vi "read_raw_data.vi"() -> ()   [LabVIEW 2017]
uses:
  <vilib>/Utility/file.llb/Write Delimited Spreadsheet (I64).vi
panel:
  out "file path (dialog if empty) 2":path
  out "ip":u64 format="%x"
  out "data 9":string
  out "result string":string
  out "sent number":u64 format="%x"
  out "trigger number":u64 format="%x"
  out "data 8":string
  out "data 7":string
  out "data":u64[](array[numeric]) format="%x"
  out "data 2":string
  out "data 4":string
  out "coarse time":u64 format="%x"
  out "error out":errorcluster
  out "substring":string
  out "number 3":u32
  out "channel number":u64 format="%x"
  in  "channel":u64
  out "data 6":string
  out "data 3":string
  in  "file (use dialog)":path
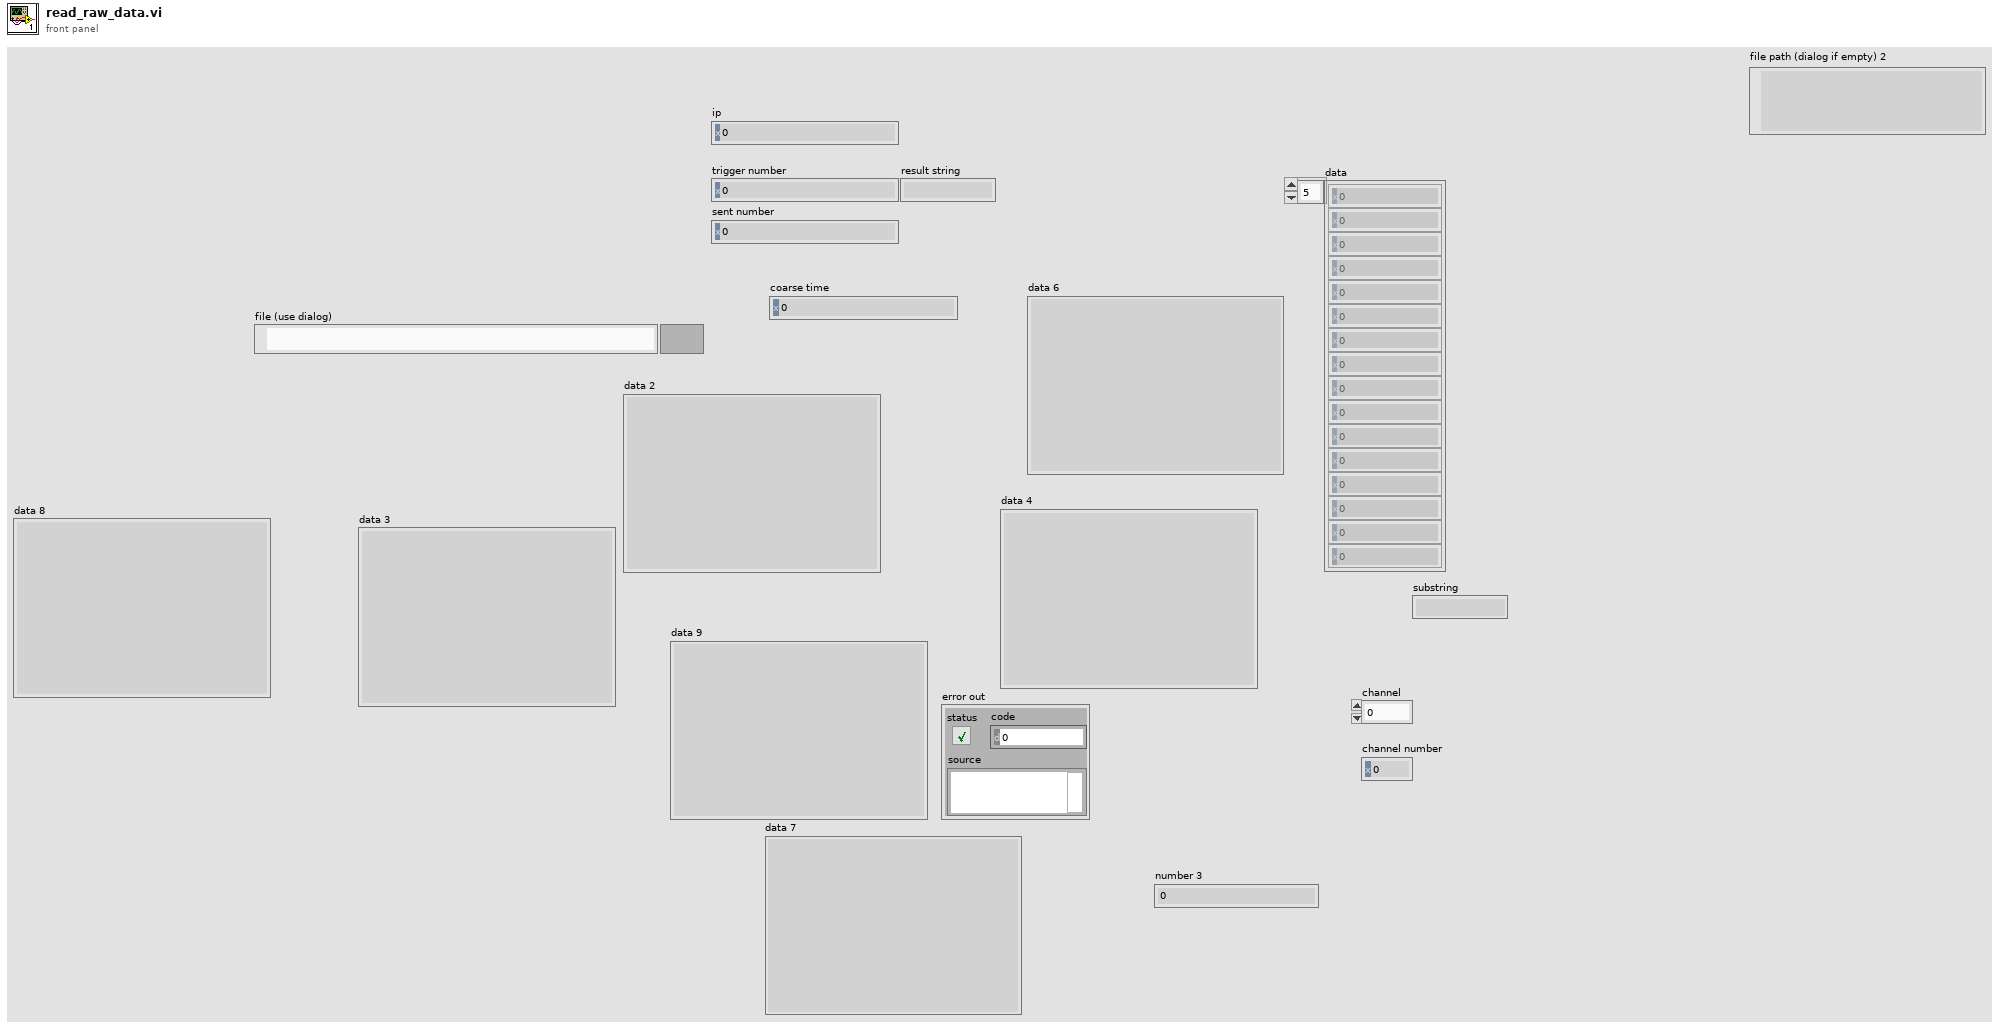
[diagram p1: front panel]
types:
  T1 = enum16{"open", "replace", "create", "open or create", "replace or create", "replace or create with confirmation"}
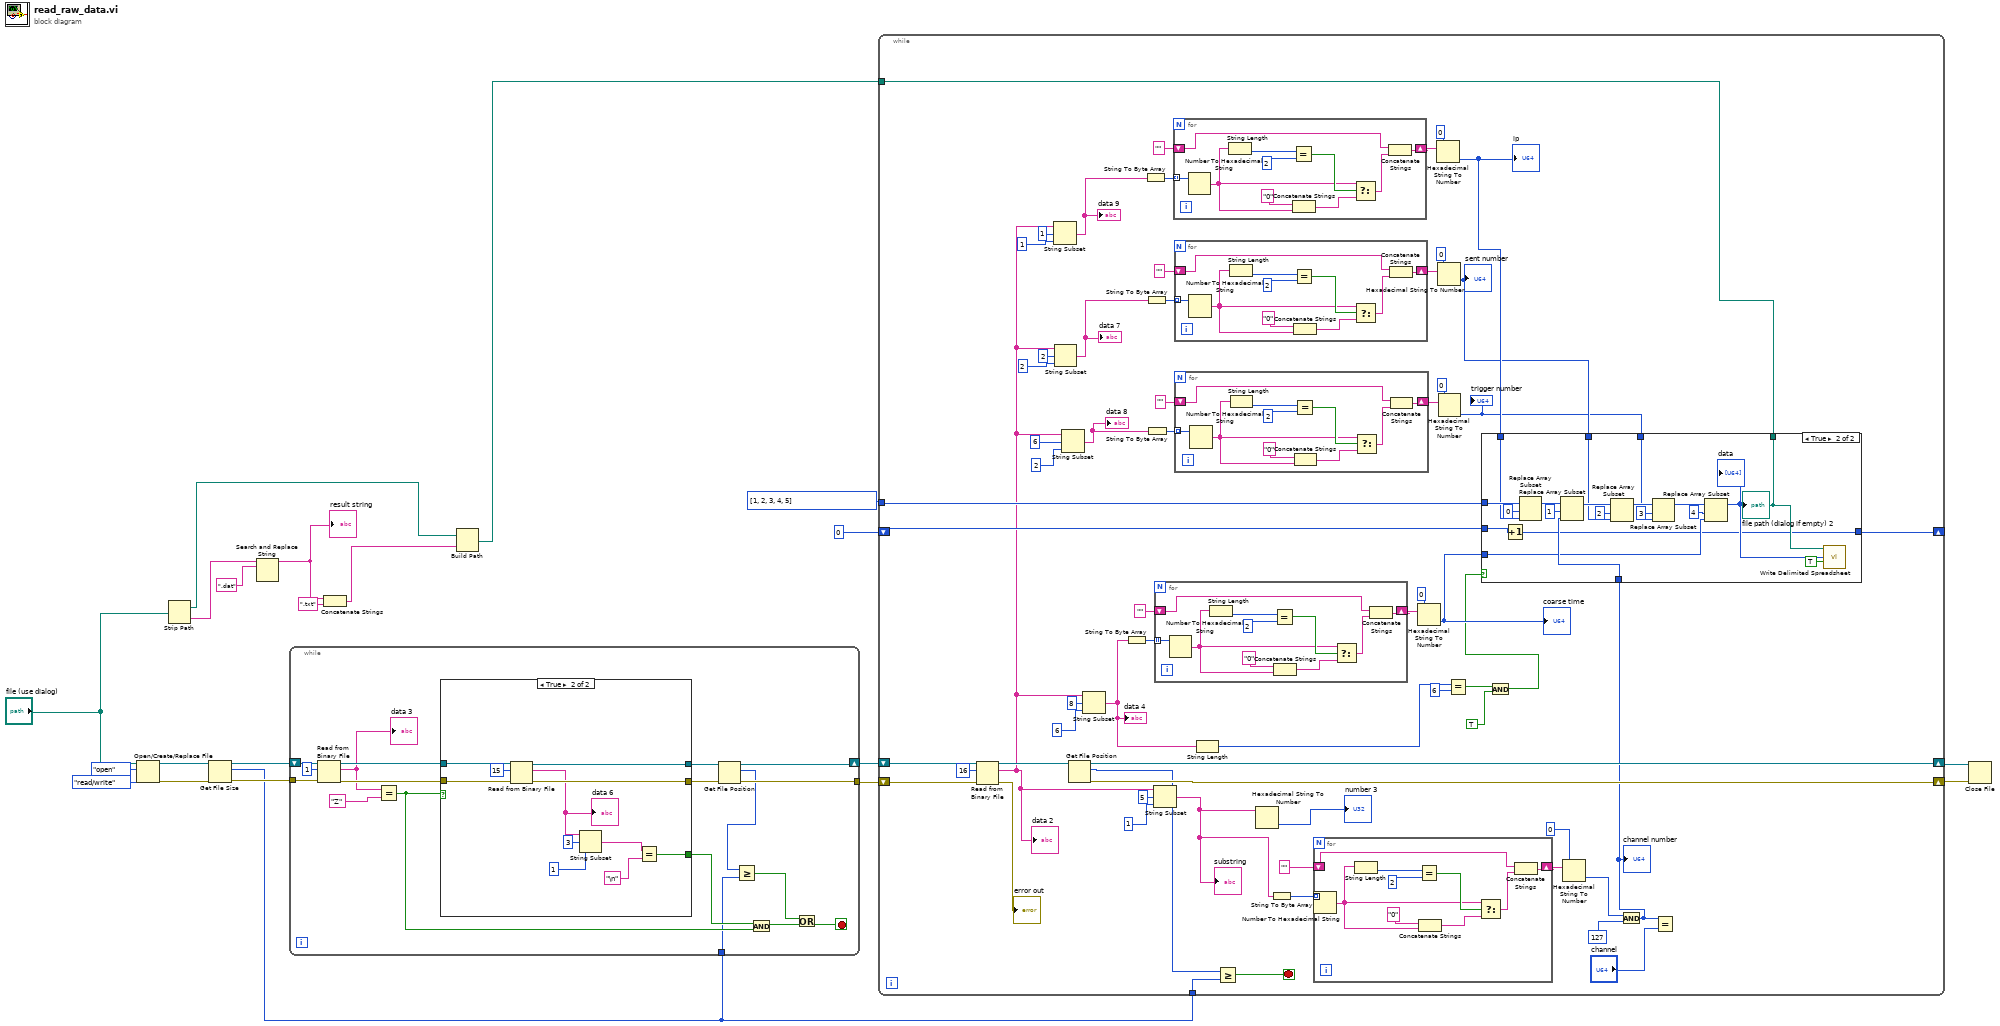
[diagram p0: block diagram]
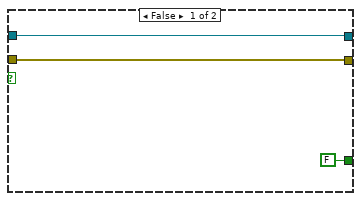
[diagram p3: hidden frame]
diagram:
  n1 = Open/Create/Replace File(file path (use dialog)="file (use dialog)", operation (0:open)=T1."open", access (0:read/write)=enum16{"read/write", "read-only", "write-only"}."read/write") -> (refnum out=w21:refnum<file>, error out=w15:errorcluster)  [unwired: 3 in, 1 out]
  n2 = Strip Path(path="file (use dialog)") -> (stripped path=w2:path, name=w7:string)
  n3 = Get File Size(file=w21, error in=w15) -> (refnum out=w16:refnum<file>, size (in bytes)=w9:i64, 0:w14:errorcluster)
  n4 = Search and Replace String(input string=w7, search string=".dat") -> (result string=w5:string)  [unwired: 6 in, 3 out]
  "result string" <- w5
  n5 = while {
    tunnel: w14 -> [w38]
    shift-right: [w26] -> w17
    shift-left: w16 -> [w39]
    tunnel: [w27] -> w18
    tunnel: w9 -> [w25]
    stop <- w23 stop-if-true
    n6 = Read from Binary File(8:w38, 10:1 ("count (1)"), 11:w39) -> (0:w34:errorcluster, 2:w32:string, 3:w35:refnum<file>)  [unwired: 3 in, 1 out]
    "data 3" <- w32
    n7 = Equal?(x=w32, y="Z") -> (x = y?=w29:bool)
    n8 = case shown="True" w29 {
      tunnel: w35 -> [w42 w53]
      tunnel: w34 -> [w41 w52]
      tunnel: [w42 w50] -> w33
      tunnel: [w41 w49] -> w28
      tunnel: [FALSE w43] -> w30
      frame False {
      }
      frame True {
        n9 = Read from Binary File(8:w52, 10:15 ("count (1)"), 11:w53) -> (0:w49:errorcluster, 2:w46:string, 3:w50:refnum<file>)  [unwired: 3 in, 1 out]
        "data 6" <- w46
        n10 = String Subset(string=w46, offset (0)=3, length (rest)=1 ("length (rest)")) -> (substring=w45:string)
        n11 = Equal?(x=w45, y="\n") -> (x = y?=w43:bool)
      }
    }
    n12 = Get File Position(4:w28, 7:w33) -> (0:w27:errorcluster, 2:w24:i64, 3:w26:refnum<file>)
    n13 = Greater Or Equal?(x=w24, y=w25) -> (x >= y?=w22:bool)
    n14 = Compound Arithmetic op=AND(w30, w29) -> (w31:bool)
    n15 = Or(x=w22, y=w31) -> (x .or. y?=w23:bool)
  }
  n16 = Concatenate Strings(w5, ".txt" ("string")) -> (w3:string)
  n17 = Build Path(base path=w2, name or relative path=w3) -> (appended path=w1:path)
  n18 = while {
    shift-right: [w112] -> w13
    shift-left: w17 -> [w116]
    shift-right: [w114] -> w12
    shift-left: w18 -> [w117]
    tunnel: w9 -> [w110]
    shift-right: [w54] -> _
    shift-left: 0 ("length (rest)") -> [w89]
    tunnel: w1 -> [w55]
    tunnel: u64[] [1, 2, 3, 4, 5] -> [w88]
    stop <- w109 stop-if-true
    n19 = Read from Binary File(8:w117, 10:16 ("count (1)"), 11:w116) -> (0:→"error out":errorcluster, 2:w60:string, 3:w113:refnum<file>)  [unwired: 3 in, 1 out]
    "data 2" <- w60
    n20 = String Subset(string=w60, offset (0)=1, length (rest)=1 ("length (rest)")) -> (substring=w67:string)
    "data 9" <- w67
    n21 = String Subset(string=w60, offset (0)=2, length (rest)=2 ("length (rest)")) -> (substring=w69:string)
    "data 7" <- w69
    n22 = String Subset(string=w60, offset (0)=6, length (rest)=2 ("length (rest)")) -> (substring=w74:string)
    "data 8" <- w74
    n23 = Get File Position(7:w113) -> (0:w114:errorcluster, 2:w111:i64, 3:w112:refnum<file>)  [unwired: 1 in]
    n24 = String Subset(string=w60, offset (0)=8, length (rest)=6 ("length (rest)")) -> (substring=w85:string)
    "data 4" <- w85
    n25 = String To Byte Array(string=w85) -> (unsigned byte array=w105:u8[])
    n26 = String To Byte Array(string=w67) -> (unsigned byte array=w64:u8[])
    n27 = String To Byte Array(string=w69) -> (unsigned byte array=w72:u8[])
    n28 = String To Byte Array(string=w74) -> (unsigned byte array=w76:u8[])
    n29 = String Subset(string=w60, offset (0)=5, length (rest)=1 ("length (rest)")) -> (substring=w92:string)
    "substring" <- w92
    n30 = for {
      shift-right: [w187] -> w104
      shift-left: "" ("format string") -> [w184]
      tunnel: w105 -> [w188] mode=indexing
      n31 = Number To Hexadecimal String(2:w188) -> (0:w180:string)  [unwired: 1 in]
      n32 = String Length(string=w180) -> (length=w186:i32)
      n33 = Equal?(x=w186, y=2) -> (x = y?=w183:bool)
      n34 = Concatenate Strings("0" ("format string"), w180) -> (w182:string)
      n35 = Select(t=w180, s=w183, f=w182) -> (s? t:f=w179:string)
      n36 = Concatenate Strings(w184, w179) -> (w187:string)
    }
    n37 = for {
      shift-right: [w126] -> w65
      shift-left: "" ("format string") -> [w123]
      tunnel: w64 -> [w127] mode=indexing
      n38 = Number To Hexadecimal String(2:w127) -> (0:w119:string)  [unwired: 1 in]
      n39 = String Length(string=w119) -> (length=w125:i32)
      n40 = Equal?(x=w125, y=2) -> (x = y?=w122:bool)
      n41 = Concatenate Strings("0" ("format string"), w119) -> (w121:string)
      n42 = Select(t=w119, s=w122, f=w121) -> (s? t:f=w118:string)
      n43 = Concatenate Strings(w123, w118) -> (w126:string)
    }
    n44 = for {
      shift-right: [w136] -> w71
      shift-left: "" ("format string") -> [w133]
      tunnel: w72 -> [w137] mode=indexing
      n45 = Number To Hexadecimal String(2:w137) -> (0:w129:string)  [unwired: 1 in]
      n46 = String Length(string=w129) -> (length=w135:i32)
      n47 = Equal?(x=w135, y=2) -> (x = y?=w132:bool)
      n48 = Concatenate Strings("0" ("format string"), w129) -> (w131:string)
      n49 = Select(t=w129, s=w132, f=w131) -> (s? t:f=w128:string)
      n50 = Concatenate Strings(w133, w128) -> (w136:string)
    }
    n51 = for {
      shift-right: [w146] -> w77
      shift-left: "" ("format string") -> [w143]
      tunnel: w76 -> [w147] mode=indexing
      n52 = Number To Hexadecimal String(2:w147) -> (0:w139:string)  [unwired: 1 in]
      n53 = String Length(string=w139) -> (length=w145:i32)
      n54 = Equal?(x=w145, y=2) -> (x = y?=w142:bool)
      n55 = Concatenate Strings("0" ("format string"), w139) -> (w141:string)
      n56 = Select(t=w139, s=w142, f=w141) -> (s? t:f=w138:string)
      n57 = Concatenate Strings(w143, w138) -> (w146:string)
    }
    n58 = String Length(string=w85) -> (length=w83:i32)
    n59 = Greater Or Equal?(x=w111, y=w110) -> (x >= y?=w109:bool)
    n60 = Hexadecimal String To Number(string=w92) -> (number=→"number 3":u32)  [unwired: 2 in, 1 out]
    n61 = String To Byte Array(string=w92) -> (unsigned byte array=w95:u8[])
    n62 = for {
      shift-right: [w177] -> w94
      shift-left: "" ("format string") -> [w174]
      tunnel: w95 -> [w178] mode=indexing
      n63 = Number To Hexadecimal String(2:w178) -> (0:w170:string)  [unwired: 1 in]
      n64 = String Length(string=w170) -> (length=w176:i32)
      n65 = Equal?(x=w176, y=2) -> (x = y?=w173:bool)
      n66 = Concatenate Strings("0" ("format string"), w170) -> (w172:string)
      n67 = Select(t=w170, s=w173, f=w172) -> (s? t:f=w169:string)
      n68 = Concatenate Strings(w174, w169) -> (w177:string)
    }
    n69 = Hexadecimal String To Number(string=w104, default (0uL)=u64 0 ("default (0 U32)")) -> (number=w87:u64)  [unwired: 1 in, 1 out]
    "coarse time" <- w87
    n70 = Hexadecimal String To Number(string=w65, default (0uL)=u64 0 ("default (0 U32)")) -> (number=w59:u64)  [unwired: 1 in, 1 out]
    "ip" <- w59
    n71 = Hexadecimal String To Number(string=w71, default (0uL)=u64 0 ("default (0 U32)")) -> (number=w58:u64)  [unwired: 1 in, 1 out]
    "sent number" <- w58
    n72 = Hexadecimal String To Number(string=w77, default (0uL)=u64 0 ("default (0 U32)")) -> (number=w57:u64)  [unwired: 1 in, 1 out]
    "trigger number" <- w57
    n73 = Equal?(x=w83, y=6) -> (x = y?=w84:bool)
    n74 = And(x=w84, y=TRUE) -> (x .and. y?=w81:bool)
    n75 = Hexadecimal String To Number(string=w94, default (0uL)=u64 0 ("default (0 U32)")) -> (number=w91:u64)  [unwired: 1 in, 1 out]
    n76 = And(x=w91, y=u64 127 ("default (0 U32)")) -> (x .and. y?=w56:u64)
    "channel number" <- w56
    n77 = case shown="True" w81 {
      tunnel: w89 -> [w148 w150]
      tunnel: w88 -> [_ w168]
      tunnel: w87 -> [_ w151]
      tunnel: w59 -> [_ w166]
      tunnel: w58 -> [_ w158]
      tunnel: w57 -> [_ w159]
      tunnel: w56 -> [_ w157]
      tunnel: w55 -> [_ w155]
      tunnel: [w148 w149] -> w54
      frame False {
      }
      frame True {
        n78 = Increment(x=w150) -> (x+1=w149:i32)
        n79 = Replace Array Subset(array=w168, new element=w166, index=0) -> (w165:u64[])
        n80 = Replace Array Subset(array=w165, new element=w157, index=1) -> (w160:u64[])
        n81 = Replace Array Subset(array=w160, new element=w158, index=2) -> (w162:u64[])
        n82 = Replace Array Subset(array=w162, new element=w159, index=3) -> (w153:u64[])
        n83 = Replace Array Subset(array=w153, new element=w151, index=4) -> (w152:u64[])
        "data" <- w152
        n84 = call-poly <vilib>:"Write Delimited Spreadsheet.vi"("file path (dialog if empty)"=w155, "1D data"=w152, "append to file? (new file:F)"=TRUE) -> ()  [unwired: 11 in, 2 out]
        "file path (dialog if empty) 2" <- w155
      }
    }
    n85 = Equal?(x=w56, y="channel") -> ()  [unwired: 1 out]
  }
  n86 = Close File(refnum=w13, error in=w12) -> ()  [unwired: 2 out]
